vi "Execute.vi"(8 "error in (no error)":errorcluster, 10 "SQL Statement in":refnum<class "SQL Statement.lvclass">) -> (0 "error out":errorcluster)   [LabVIEW 2015, in "DBToolkit.lvlib"]
uses:
  DBToolkit.lvlib
  <vilib>/drjdpowell/SQLite Library/SQL Statement/SQL Statement.lvclass
  <vilib>/drjdpowell/SQLite Library/SQL Statement/SQL Statement.lvclass/SQL Statement.ctl
  <vilib>/drjdpowell/SQLite Library/SQL Statement/Step.vi
  <vilib>/drjdpowell/SQLite Library/SQL Statement/Error Message.vi
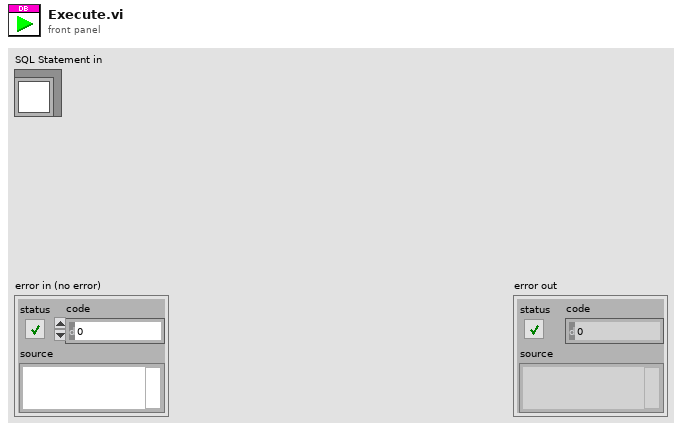
[diagram p1: front panel]
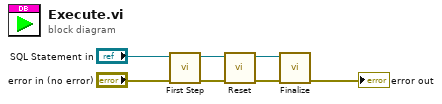
[diagram p0: block diagram]
diagram:
  n1 = call <vilib>:"First Step.vi"("error in (no error)"="error in (no error)", "SQL Statement in"="SQL Statement in") -> ("error out"=w6:errorcluster, "SQL Statement out"=w7:refnum<class "SQL Statement.lvclass">)  [unwired: 7 in, 1 out]
  n2 = call <vilib>:"Reset.vi"("error in (no error)"=w6, "SQL Statement in"=w7) -> ("error out"=w4:errorcluster, "SQL Statement out"=w5:refnum<class "SQL Statement.lvclass">)  [unwired: 8 in]
  n3 = call <vilib>:"Finalize.vi"("error in (no error)"=w4, "SQL Statement in"=w5) -> ("error out"=→"error out":errorcluster)  [unwired: 9 in]
